vi "Aero_tunnel_monitor.vi"() -> ()   [LabVIEW 2013]
uses:
  Controls/Post_Process.ctl
  <vilib>/Platform/TimedLoop/XDataNode/timing_clust.ctl
  <vilib>/Platform/TimedLoop/XDataNode/nitl_modes.ctl
  <vilib>/Platform/TimedLoop/XDataNode/wakeup.ctl
  ADAM Client/Sub VIs/ADAM Controls/Update_scan_value.ctl
  Globals/Meas_global.vi
  <vilib>/Platform/TimedLoop/XDataNode/XDataNode.xnode
  <vilib>/Platform/TimedLoop/XDataNode/XDNodeRunTimeDep.lvlib
panel:
  in  "Display Graph?":bool
  in  "Menu Ring":u16(ring) items=["Lift", "Pitch", "Drag", "Side", "Yaw", "Roll"]
  in  "Samples":i32=1000
  out "Waveform Chart":dbl[](graph)
  in  "Output Roll":bool
  out "Roll":string="0.0 Nm"
  in  "Output Yaw":bool
  out "Yaw":string="0.0 Nm"
  in  "Output Pitch":bool
  out "Pitch":string="0.0 Nm"
  in  "Output SF":bool
  out "SF":string="0.0 N"
  in  "Output Drag":bool
  out "Drag":string="0.0 N"
  in  "Output Lift":bool
  out "Lift":string="0.0 N"
  in  "Balance Safety limits":T1(array[cluster])=[{"Max +ve Range"=80, "Max -ve Range"=80, "Axis"="Lift"}, {"Max +ve Range"=80, "Max -ve Range"=80, "Axis"="Pitch"}, {"Max +ve Range"=80, "Max -ve Range"=80, "Axis"="Drag"}, {"Max +ve Range"=80, "Max -ve Range"=80, "Axis"="Side-Force"}, {"Max +ve Range"=99, "Max -ve Range"=99, "Axis"="Yaw"}, {"Max +ve Range"=80, "Max -ve Range"=80, "Axis"="Roll"}] {"Max -ve Range" min=0 max=125; "Max +ve Range" min=0 max=125}
  out "Monitor Speed (Hz)":dbl
  out "Belt slip warning":bool
  out "Road Status":string="???"
  in  "GotoYaw":bool
  in  "NewYawPos":dbl
  out "YAW POSITION":dbl
  out "Required WindSpeedRatio":dbl
  out "ROAD SPEED m/s":dbl
  in  "BL Fan1":i32
  in  "BL Fan2":i32
  in  "Stop drive":bool
  in  "Start Drive":bool
  in  "Synch to Wind":bool
  out "Road Info":string="???"
  in  "stop":bool
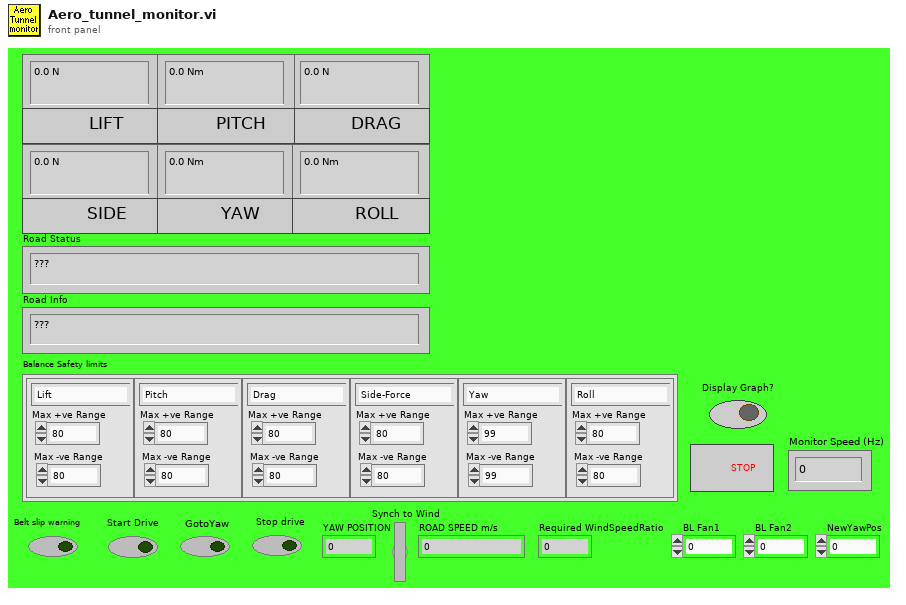
[diagram p1: front panel]
types:
  T1 = cluster{"Max +ve Range":i32, "Max -ve Range":i32, "Axis":string}[]
  T2 = typedef "Post_Process.ctl" = enum16{"Take New Data", "Post Process Raw Data File"}
  T3 = typedef "XDNodeRunTimeDep.lvlib/timing_clust.ctl" = cluster{"Expected End [f-1]":u64, "Actual End [f-1]":u64, "Finished Late? [f-1]":bool, "Expected End [i-1]":u64, "Actual End [i-1]":u64, "Finished Late? [i-1]":bool, "Expected Start [i]":u64, "Actual Start [i]":u64, "Expected Start [f]":u64, "Actual Start [f]":u64, "Source Name":string, "Structure Name":string, "Period":i64, "Deadline":i64, "Offset":i64, "Start":i64, "Priority":i32, "Timeout":i32, "Mode":T4, "Wakeup Reason":T5, "Error":errorcluster, "Source Type":string, "Secondary Source Type":string, "Global End Time":u64, "Global Start Time":u64, "Frame Duration":u64, "Iteration Duration":u64, "Assigned CPU":i32, "I/O Scan Engine Mode":u32}
  T4 = typedef "XDNodeRunTimeDep.lvlib/nitl_modes.ctl" = enum32{"No Change", "Process missed periods, maintain original phase", "Discard missed periods, maintain original phase", "Process missed periods, ignore original phase", "Discard missed periods, ignore original phase"}
  T5 = typedef "XDNodeRunTimeDep.lvlib/wakeup.ctl" = enum32{"Normal", "Aborted", "Asynchronous wakeup", "Timing source error", "Timed loop error", "Timeout"}
  T6 = typedef "Update_scan_value.ctl" = cluster{"Channel Name":string, "New Value":dbl}
  T7 = cluster{"Max +ve Range":i32, "Max -ve Range":i32, "Axis":string}
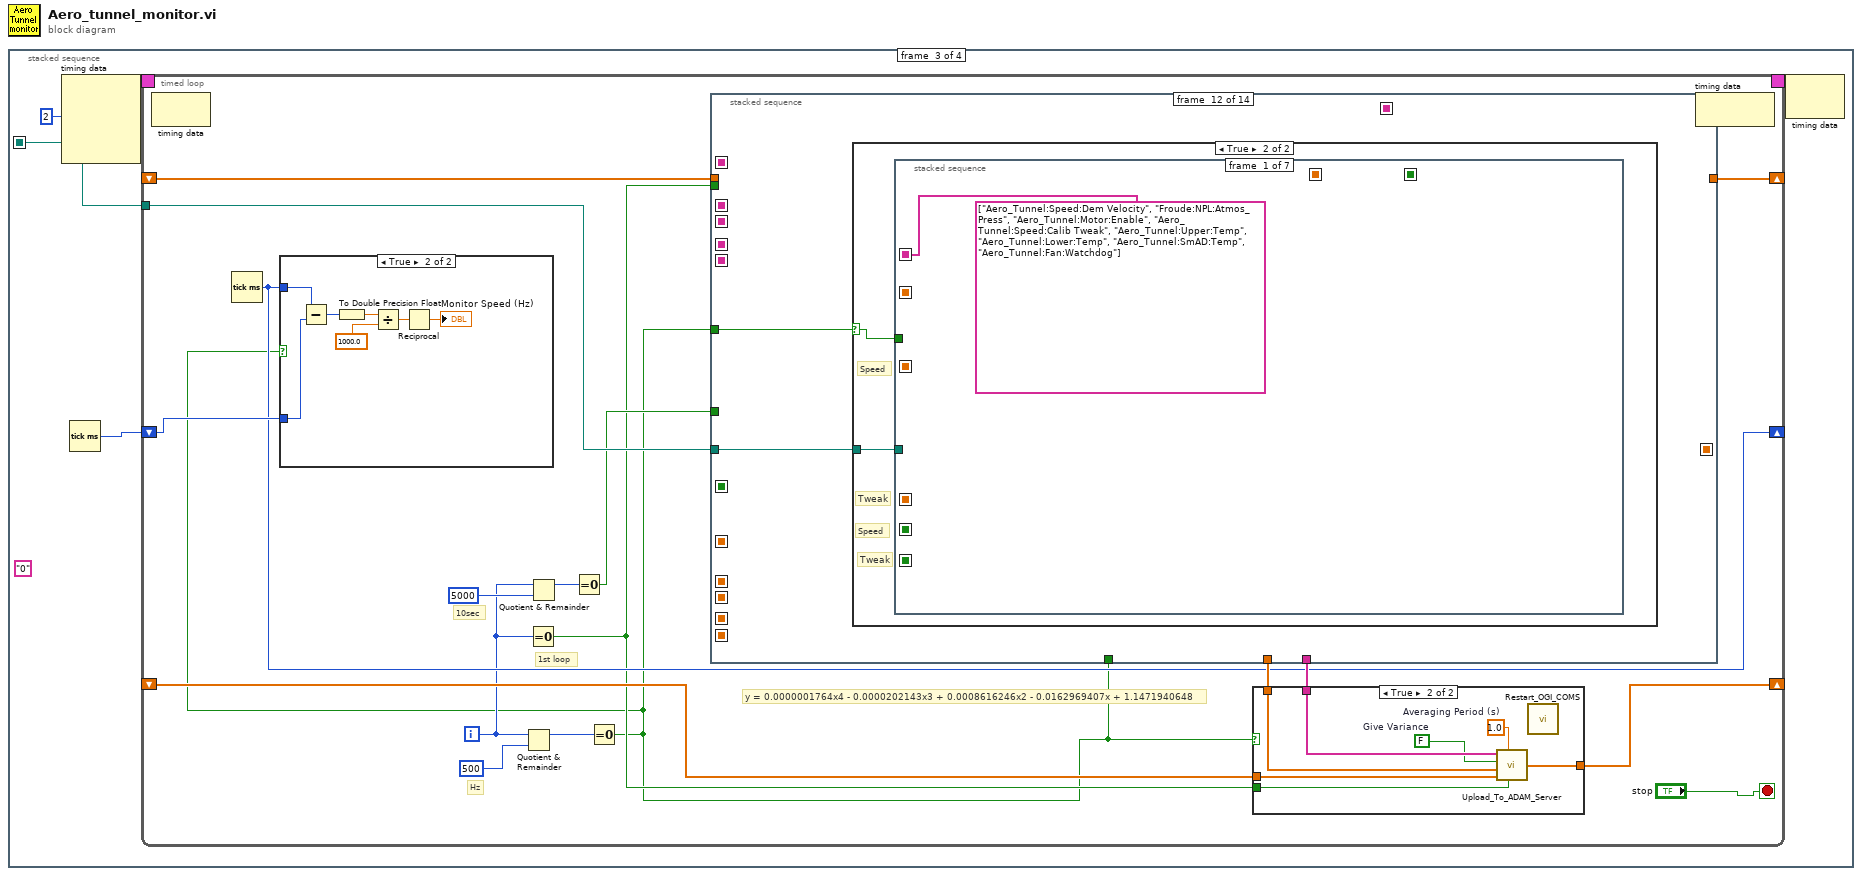
[diagram p0: block diagram]
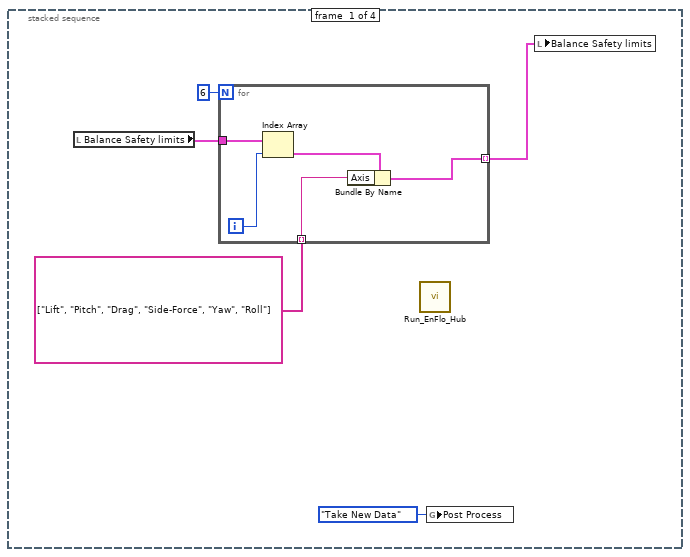
[diagram p2: hidden frame]
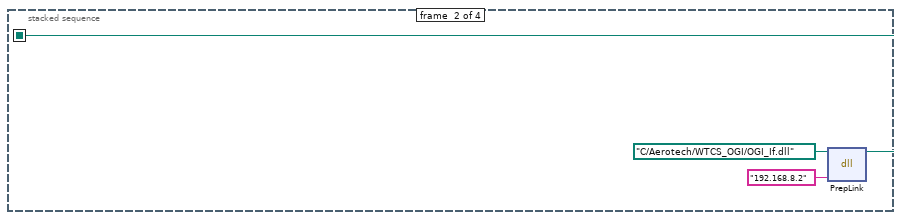
[diagram p3: hidden frame]
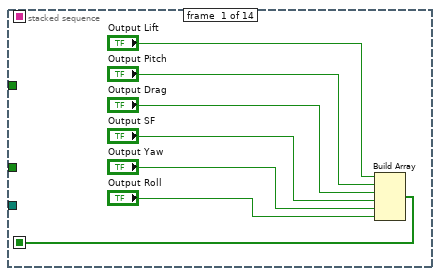
[diagram p6: hidden frame]
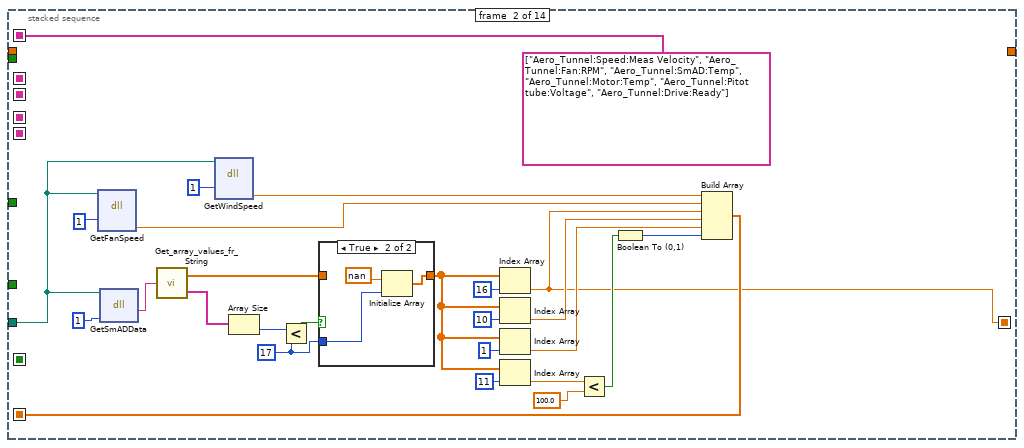
[diagram p7: hidden frame]
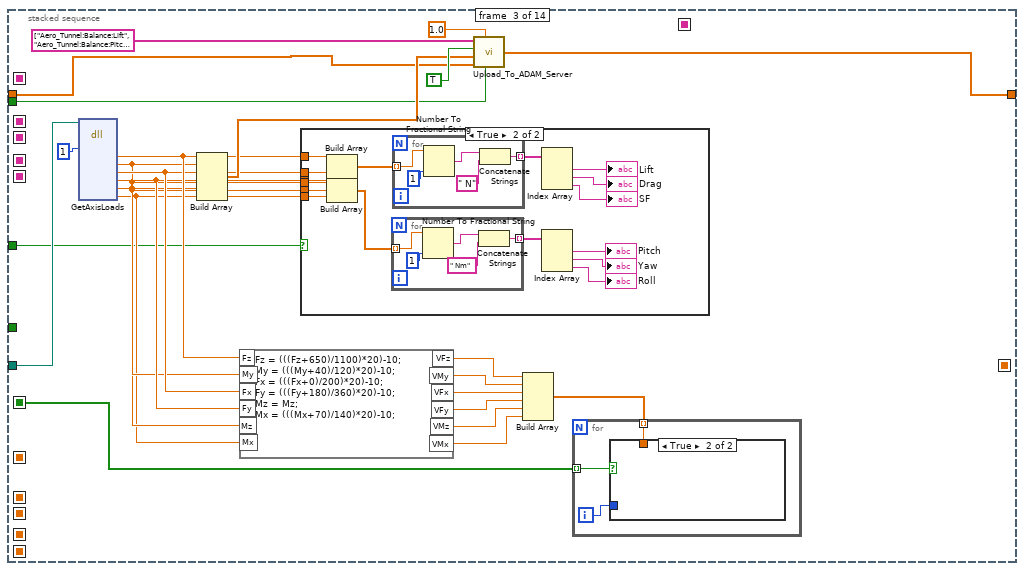
[diagram p9: hidden frame]
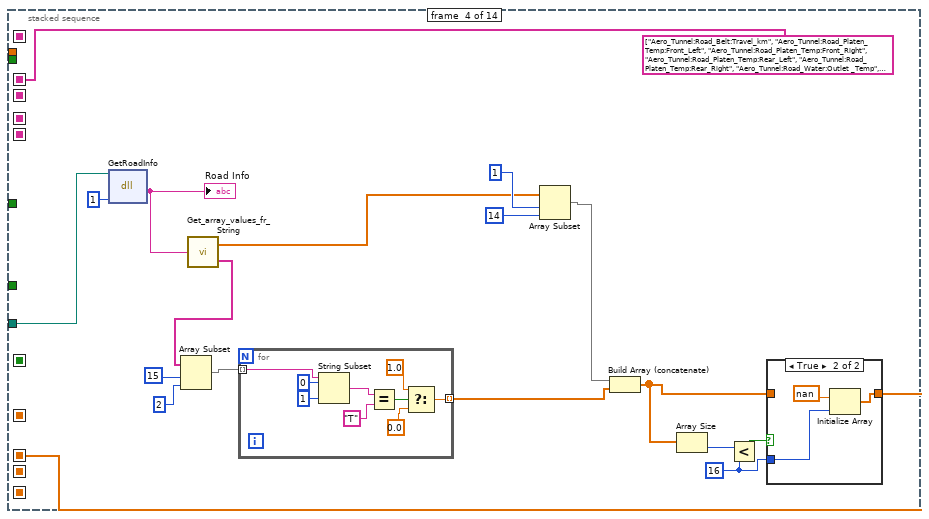
[diagram p12: hidden frame]
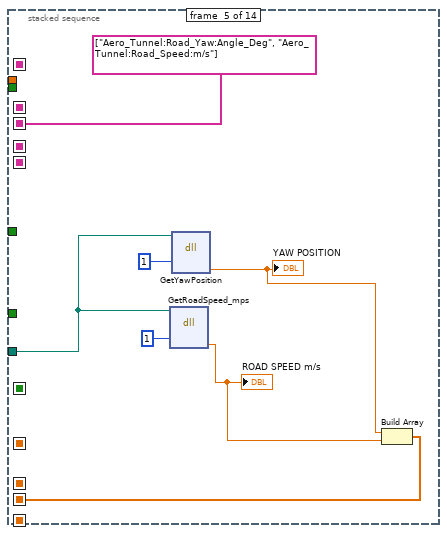
[diagram p14: hidden frame]
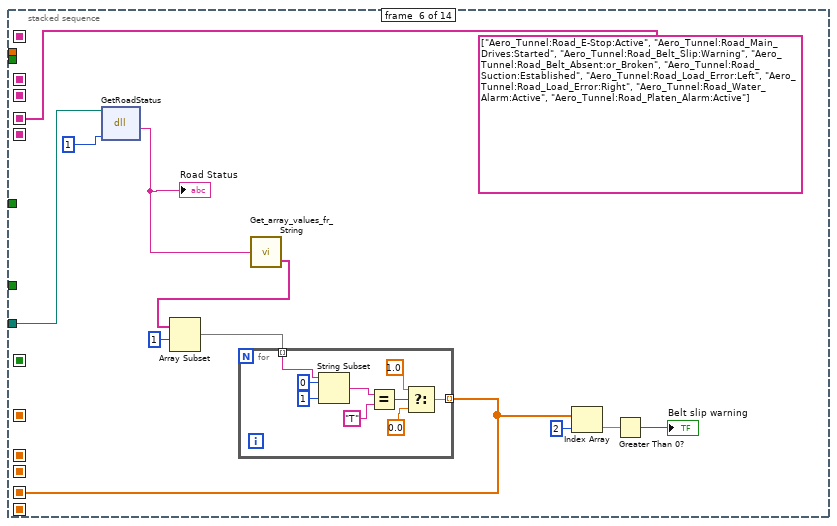
[diagram p15: hidden frame]
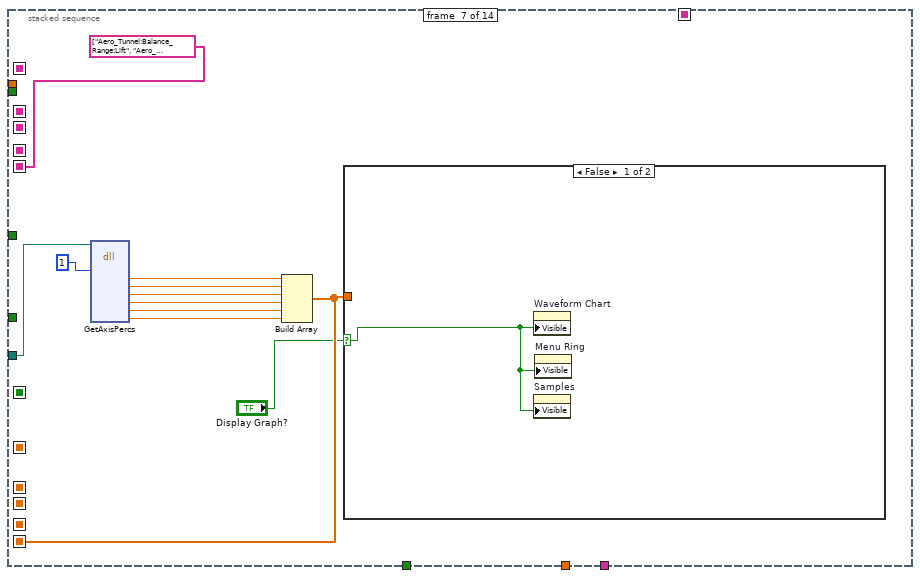
[diagram p16: hidden frame]
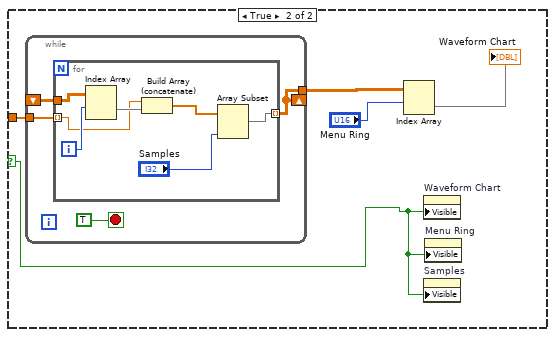
[diagram p17: hidden frame]
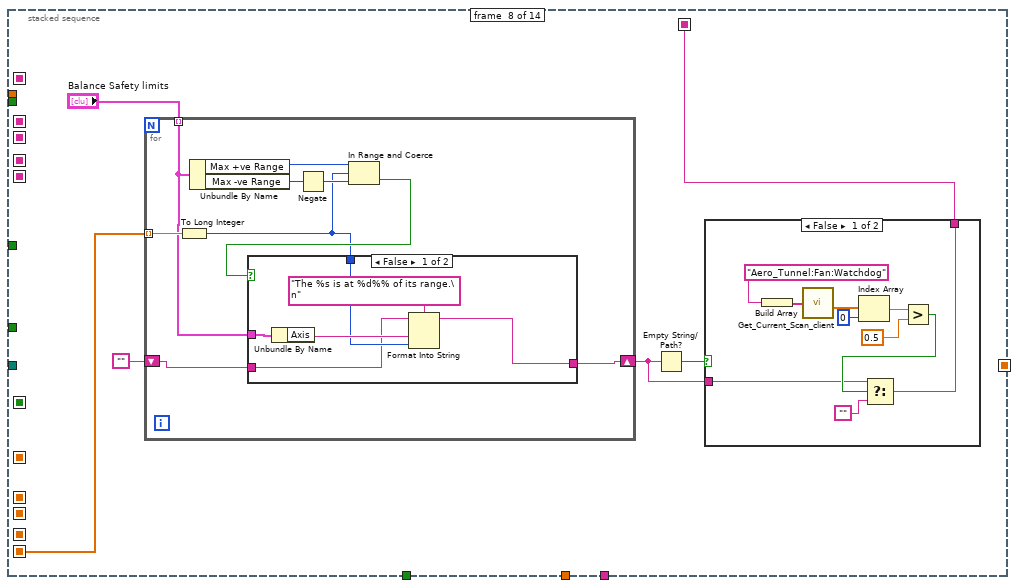
[diagram p18: hidden frame]
diagram:
  n1 = stacked-sequence {
    seq-local: [_ w11 _ _] -> [_ _ w18 w519]
    frame #0 {
      n2 = local read "Balance Safety limits"() -> (w4:T1)
      n3 = for {
        N: 6 -> [_]
        tunnel: w4 -> [w10]
        tunnel: [w7] -> w3 mode=indexing
        tunnel: string[] ["Lift", "Pitch", "Drag", "Side-Force", "Yaw", "Roll"] ("Channel Names") -> [w6] mode=indexing
        i -> [w9]
        n4 = Index Array(array=w10, index=w9) -> (element=w8:T7)
        n5 = Bundle By Name(cluster=w8, "Axis"=w6) -> (w7:T7)
      }
      n6 = call "Run_EnFlo_Hub.vi"() -> ()  [unwired: 8 in]
      n7 = global write "Meas_global.vi" "Post Process"(Post_Process."Take New Data" ("Post Process")) -> ()
      n8 = local write "Balance Safety limits"(w3) -> ()
    }
    frame #1 {
      n9 = dll-call lib="C:/Aerotech/Drivers/OGI_IF.dll" fn="PrepLink"(path in=path "C:/Aerotech/WTCS_OGI/OGI_If.dll", "IPAddress"="192.168.8.2") -> (path out=w11:path)  [unwired: 2 in, 3 out]
    }
    frame #2 {
      (unwired) "0" ("Channels")
      n10 = node-c288(i64 2 ("Period")) -> (w16:T3)  [unwired: 3 in]
      n11 = Tick Count (ms)() -> (millisecond timer value=w17:u32)
      n12 = timed-loop {
        shift-right: [w36] -> _
        shift-left: _ -> [w34]
        tunnel: w18 -> [w32]
        shift-right: [w30] -> _
        shift-left: _ -> [w31]
        timing: w16 -> [_]
        timing-out: [_] -> w15
        shift-right: [w28] -> _
        shift-left: w17 -> [w29]
        i -> [w22]
        stop <- "stop" stop-if-true
        # "1st loop"
        # "10sec"
        # "Hz"
        # "y = 0.0000001764x4 - 0.0000202143x3 + 0.0008616246x2 - 0.0162969407x + 1.1471940648"
        n13 = node-c288() -> ()  [unwired: 1 in, 1 out]
        n14 = Tick Count (ms)() -> (millisecond timer value=w28:u32)
        n15 = Quotient & Remainder(x=w22, y=500) -> (x-y*floor(x/y)=w25:i32)  [unwired: 1 out]
        n16 = Equal To 0?(x=w22) -> (x = 0?=w21:bool)
        n17 = Quotient & Remainder(x=w22, y=5000) -> (x-y*floor(x/y)=w24:i32)  [unwired: 1 out]
        n18 = Equal To 0?(x=w24) -> (x = 0?=w23:bool)
        n19 = Equal To 0?(x=w25) -> (x = 0?=w20:bool)
        n20 = case shown="True" w20 {
          tunnel: w29 -> [_ w43]
          tunnel: w28 -> [_ w42]
          frame False {
          }
          frame True {
            n21 = Subtract(x=w42, y=w43) -> (x-y=w41:u32)
            n22 = To Double Precision Float(number=w41) -> (double precision float=w37:dbl)
            n23 = Divide(x=w37, y=1000.0) -> (x/y=w39:dbl)
            n24 = Reciprocal(x=w39) -> (1/x=→"Monitor Speed (Hz)":dbl)
          }
        }
        n25 = stacked-sequence {
          seq-local: [_ string[] ["Aero_Tunnel:Speed:Meas Velocity", "Aero_Tunnel:Fan:RPM", "Aero_Tunnel:SmAD:Temp", "Aero_Tunnel:Motor:Temp", "Aero_Tunnel:Pitot tube:Voltage", "Aero_Tunnel:Drive:Ready"] ("Channel Names") _ _ _ _ _ _ _ _ _ _ _ _] -> [_ _ _ _ _ _ _ _ _ _ w319 _ _ _]
          seq-local: [_ w76 _ _ _ _ _ _ _ _ _ _ _ _] -> [_ _ _ _ _ _ _ _ _ _ w318 _ _ _]
          seq-local: [_ _ _ w144 _ _ _ _ _ _ _ _ _ _] -> [_ _ _ _ _ _ _ _ _ _ w315 _ _ _]
          seq-local: [_ _ _ string[] ["Aero_Tunnel:Road_Belt:Travel_km", "Aero_Tunnel:Road_Platen_Temp:Front_Left", "Aero_Tunnel:Road_Platen_Temp:Front_Right", "Aero_Tunnel:Road_Platen_Temp:Rear_Left", "Aero_Tunnel:Road_Platen_Temp:Rear_Right", "Aero_Tunnel:Road_Water:Outlet _Temp", "Aero_Tunnel:Road_Water:Inlet _Temp", "Aero_Tunnel:Road_Suction:Front", "Aero_Tunnel:Road_Suction:Middle", "Aero_Tunnel:Road_Suction:Rear", "Aero_Tunnel:Road_BL_Suction:Primary", "Aero_Tunnel:Road_BL_Suction:Secondary", "Aero_Tunnel:Road_LoadCell:Left", "Aero_Tunnel:Road_LoadCell:Right", "Aero_Tunnel:Road_Water_High:Temp_Alarm", "Aero_Tunnel:Road_Platen_High:Temp_Alarm"] ("Channel Names") _ _ _ _ _ _ _ _ _ _] -> [_ _ _ _ _ _ _ _ _ _ w304 _ _ _]
          seq-local: [_ _ _ _ string[] ["Aero_Tunnel:Road_Yaw:Angle_Deg", "Aero_Tunnel:Road_Speed:m/s"] ("Channel Names") _ _ _ _ _ _ _ _ _] -> [_ _ _ _ _ _ _ _ _ _ w314 _ _ _]
          seq-local: [_ _ _ _ w175 _ _ _ _ _ _ _ _ _] -> [_ _ _ _ _ _ _ _ _ _ w313 _ _ _]
          seq-local: [_ _ _ _ _ string[] ["Aero_Tunnel:Road_E-Stop:Active", "Aero_Tunnel:Road_Main_Drives:Started", "Aero_Tunnel:Road_Belt_Slip:Warning", "Aero_Tunnel:Road_Belt_Absent:or_Broken", "Aero_Tunnel:Road_Suction:Established", "Aero_Tunnel:Road_Load_Error:Left", "Aero_Tunnel:Road_Load_Error:Right", "Aero_Tunnel:Road_Water_Alarm:Active", "Aero_Tunnel:Road_Platen_Alarm:Active"] ("Channel Names") _ _ _ _ _ _ _ _] -> [_ _ _ _ _ _ _ _ _ _ w309 _ _ _]
          seq-local: [_ _ _ _ _ w188 _ _ _ _ _ _ _ _] -> [_ _ _ _ _ _ _ _ _ _ w308 _ _ _]
          seq-local: [w54 _ _ _ _ _ _ _ _ _ _ _ _ _] -> [_ _ w106 _ _ _ _ _ _ _ _ _ _ _]
          seq-local: [_ _ _ _ _ _ string[] ["Aero_Tunnel:Balance_Range:Lift", "Aero_Tunnel:Balance_Range:Pitch", "Aero_Tunnel:Balance_Range:Drag", "Aero_Tunnel:Balance_Range:Side-Force", "Aero_Tunnel:Balance_Range:Yaw", "Aero_Tunnel:Balance_Range:Roll"] ("Channel Names") _ _ _ _ _ _ _] -> [_ _ _ _ _ _ _ _ _ _ w305 _ _ _]
          seq-local: [_ _ _ _ _ _ w203 _ _ _ _ _ _ _] -> [_ _ _ _ _ _ _ w234 _ _ w306 _ _ _]
          seq-local: [_ _ _ _ _ _ _ w230 _ _ _ _ _ _] -> [_ _ _ _ _ _ _ _ w264 w283 _ _ _ _]
          seq-local: [_ w61 _ _ _ _ _ _ _ _ _ _ _ _] -> [_ _ _ _ _ _ _ _ _ w282 _ _ _ _]
          tunnel: [_ _ _ _ _ _ _ _ _ _ w317 _ _ _] -> w35
          tunnel: [_ _ _ _ _ _ _ _ _ _ w316 _ _ _] -> w33
          tunnel: w32 -> [_ w68 w113 w160 w178 w191 w212 _ _ _ w307 w321 w428 w455]
          tunnel: w20 -> [_ _ _ _ _ _ _ _ _ _ _ _ _ _]
          tunnel: w31 -> [_ _ w100 _ _ _ _ _ _ _ _ _ _ _]
          tunnel: [_ _ w99 _ _ _ _ _ _ _ _ _ _ _] -> w30
          tunnel: w20 -> [_ _ w92 _ _ _ _ _ _ _ _ w320 _ w454]
          tunnel: w23 -> [_ _ _ _ _ _ _ _ w263 _ _ _ w427 _]
          tunnel: w21 -> [_ _ w91 _ _ _ _ _ _ _ _ _ _ _]
          frame #0 {
            n26 = Build Array("Output Lift", "Output Pitch", "Output Drag", "Output SF", "Output Yaw", "Output Roll") -> (w54:bool[])
          }
          frame #1 {
            w62 = 17 ("y")
            n27 = dll-call lib="C:/Aerotech/Drivers/OGI_IF.dll" fn="GetFanSpeed"(path in=w68, "Enable"=1) -> ("FanSpeedinRPM"=w70:dbl)  [unwired: 3 in, 4 out]
            n28 = dll-call lib="C:/Aerotech/Drivers/OGI_IF.dll" fn="GetSmADData"(path in=w68, "Enable"=1) -> ("SmAD Data String"=w73:string)  [unwired: 2 in, 3 out]
            n29 = call "Get_array_values_fr_String.vi"("String Value"=w73) -> ("Numeric Array"=w63:dbl[], "String array"=w66:string[])
            n30 = dll-call lib="C:/Aerotech/Drivers/OGI_IF.dll" fn="GetWindSpeed"(path in=w68, "Enable"=1) -> ("Windspeed_M/s"=w69:dbl)  [unwired: 3 in, 4 out]
            n31 = Array Size(array=w66) -> (size(s)=w67:i32)
            n32 = Less?(x=w67, y=w62) -> (x < y?=w65:bool)
            n33 = case shown="True" w65 {
              tunnel: [w87 w90] -> w64
              tunnel: w63 -> [w87 _]
              tunnel: w62 -> [_ w88]
              frame False {
              }
              frame True {
                n34 = Initialize Array(nan, w88) -> (w90:dbl[])
              }
            }
            n35 = Index Array(array=w64, index=16) -> (element=w61:dbl)
            n36 = Index Array(array=w64, index=10) -> (element=w84:dbl)
            n37 = Index Array(array=w64, index=1) -> (element=w82:dbl)
            n38 = Index Array(array=w64, index=11) -> (element=w80:dbl)
            n39 = Less?(x=w80, y=100.0) -> (x < y?=w78:bool)
            n40 = Boolean To (0,1)(Boolean=w78) -> (0, 1=w77:i16)
            n41 = Build Array(w69, w70, w61, w84, w82, w77) -> (w76:dbl[])
          }
          frame #2 {
            n42 = dll-call lib="C:/Aerotech/Drivers/OGI_IF.dll" fn="GetAxisLoads"(path in=w113, "Enable"=1) -> ("Lift"=w98:dbl, "Pitch"=w95:dbl, "Drag"=w97:dbl, "side"=w96:dbl, "Yaw"=w94:dbl, "Roll"=w93:dbl)  [unwired: 3 in, 9 out]
            n43 = Build Array(w98, w95, w97, w96, w94, w93) -> (w101:dbl[])
            n44 = formula code="VFz = (((Fz+650)/1100)*20)-10;\nVMy = (((My+40)/120)*20)-10;\nVFx = (((Fx+0)/200)*20)-10;\nVFy = (((Fy+180)/360)*20)-10;\nVMz = Mz;\nVMx = (((Mx+70)/140)*20)-10;"("Fz"=w98, "My"=w95, "Fx"=w97, "Fy"=w96, "Mz"=w94, "Mx"=w93) -> ("VFz"=w112:dbl, "VMy"=w111:dbl, "VFx"=w110:dbl, "VFy"=w109:dbl, "VMz"=w108:dbl, "VMx"=w107:dbl)
            n45 = case shown="True" w92 {
              tunnel: w98 -> [_ w130]
              tunnel: w97 -> [_ w129]
              tunnel: w96 -> [_ w128]
              tunnel: w95 -> [_ w122]
              tunnel: w94 -> [_ w121]
              tunnel: w93 -> [_ w120]
              frame False {
              }
              frame True {
                n46 = Build Array(w130, w129, w128) -> (w127:dbl[])
                n47 = Build Array(w122, w121, w120) -> (w119:dbl[])
                n48 = for {
                  tunnel: w119 -> [w131] mode=indexing
                  tunnel: [w135] -> w118 mode=indexing
                  n49 = Number To Fractional String(number=w131, precision (6)=i16 1) -> (F-format string=w132:string)  [unwired: 2 in]
                  n50 = Concatenate Strings(w132, " Nm" ("string")) -> (w135:string)
                }
                n51 = for {
                  tunnel: w127 -> [w136] mode=indexing
                  tunnel: [w140] -> w126 mode=indexing
                  n52 = Number To Fractional String(number=w136, precision (6)=i16 1) -> (F-format string=w137:string)  [unwired: 2 in]
                  n53 = Concatenate Strings(w137, " N" ("string")) -> (w140:string)
                }
                n54 = Index Array(array=w126) -> (element #1=→"Lift":string, element #2=→"Drag":string, element #3=→"SF":string)  [unwired: 3 in]
                n55 = Index Array(array=w118) -> (element #1=→"Pitch":string, element #2=→"Yaw":string, element #3=→"Roll":string)  [unwired: 3 in]
              }
            }
            n56 = call "Upload_To_ADAM_Server.vi"("First Loop"=w91, "Averaging Period (s)"=1.0, "Shift In"=w100, "Channel Values"=w101, "Give Variance"=TRUE, "Channel Names"=string[] ["Aero_Tunnel:Balance:Lift", "Aero_Tunnel:Balance:Pitch", "Aero_Tunnel:Balance:Drag", "Aero_Tunnel:Balance:Side-Force", "Aero_Tunnel:Balance:Yaw", "Aero_Tunnel:Balance:Roll"]) -> ("Shift Out"=w99:dbl[])
            n57 = Build Array(w112, w111, w110, w109, w108, w107) -> (w105:dbl[])
            n58 = for {
              tunnel: w106 -> [w143] mode=indexing
              tunnel: w105 -> [w142] mode=indexing
              i -> [w141]
              n59 = case shown="True" w143 {
                tunnel: w142 -> [_ _]
                tunnel: w141 -> [_ _]
                frame False {
                }
                frame True {
                }
              }
            }
          }
          frame #3 {
            w147 = 16 ("y")
            n60 = dll-call lib="C:/Aerotech/Drivers/OGI_IF.dll" fn="GetRoadInfo"(path in=w160, "Enable"=1) -> ("Road Info"=w159:string)  [unwired: 3 in, 2 out]
            "Road Info" <- w159
            n61 = call "Get_array_values_fr_String.vi"("String Value"=w159) -> ("Numeric Array"=w146:dbl[], "String array"=w150:string[])
            n62 = Array Subset(array=w150, index=15, length=2) -> (w154:string[])
            n63 = for {
              tunnel: w154 -> [w172] mode=indexing
              tunnel: [w166] -> w153 mode=indexing
              n64 = String Subset(string=w172, offset (0)=0, length (rest)=1 ("length (rest)")) -> (substring=w171:string)
              n65 = Equal?(x=w171, y="T") -> (x = y?=w169:bool)
              n66 = Select(t=1.0, s=w169, f=0.0) -> (s? t:f=w166:dbl)
            }
            n67 = Array Subset(array=w146, index=1, length=14) -> (w152:dbl[])
            n68 = Build Array (concatenate)(w152, w153) -> (w145:dbl[])
            n69 = Array Size(array=w145) -> (size(s)=w149:i32)
            n70 = Less?(x=w149, y=w147) -> (x < y?=w148:bool)
            n71 = case shown="True" w148 {
              tunnel: [w162 w165] -> w144
              tunnel: w145 -> [w162 _]
              tunnel: w147 -> [_ w163]
              frame False {
              }
              frame True {
                n72 = Initialize Array(nan, w163) -> (w165:dbl[])
              }
            }
          }
          frame #4 {
            n73 = dll-call lib="C:/Aerotech/Drivers/OGI_IF.dll" fn="GetRoadSpeed_mps"(path in=w178, "Enable"=1) -> ("RoadSpeed_mps"=w176:dbl)  [unwired: 3 in, 4 out]
            "ROAD SPEED m/s" <- w176
            n74 = dll-call lib="C:/Aerotech/Drivers/OGI_IF.dll" fn="GetYawPosition"(path in=w178, "Enable"=1) -> ("Yaw Position"=w177:dbl)  [unwired: 3 in, 4 out]
            "YAW POSITION" <- w177
            n75 = Build Array(w177, w176) -> (w175:dbl[])
          }
          frame #5 {
            n76 = dll-call lib="C:/Aerotech/Drivers/OGI_IF.dll" fn="GetRoadStatus"(path in=w191, "Enable"=1) -> ("Road Status"=w190:string)  [unwired: 3 in, 2 out]
            "Road Status" <- w190
            n77 = call "Get_array_values_fr_String.vi"("String Value"=w190) -> ("String array"=w184:string[])  [unwired: 1 out]
            n78 = Array Subset(array=w184, index=1) -> (w182:string[])  [unwired: 1 in]
            n79 = for {
              tunnel: [w194] -> w188 mode=indexing
              tunnel: w182 -> [w193] mode=indexing
              n80 = String Subset(string=w193, offset (0)=0, length (rest)=1 ("length (rest)")) -> (substring=w199:string)
              n81 = Equal?(x=w199, y="T") -> (x = y?=w197:bool)
              n82 = Select(t=1.0, s=w197, f=0.0) -> (s? t:f=w194:dbl)
            }
            n83 = Index Array(array=w188, index=2) -> (element=w186:dbl)
            n84 = Greater Than 0?(x=w186) -> (x > 0?=→"Belt slip warning":bool)
          }
          frame #6 {
            n85 = dll-call lib="C:/Aerotech/Drivers/OGI_IF.dll" fn="GetAxisPercs"(path in=w212, "Enable"=1) -> ("Lift"=w210:dbl, "Pitch"=w209:dbl, "Drag"=w208:dbl, "side"=w207:dbl, "Yaw"=w206:dbl, "Roll"=w205:dbl)  [unwired: 3 in, 9 out]
            n86 = Build Array(w210, w209, w208, w207, w206, w205) -> (w203:dbl[])
            n87 = case shown="False" "Display Graph?" {
              selector: "Display Graph?" -> [w213 w214]
              tunnel: w203 -> [_ w218]
              frame False {
                n88 = property on="Waveform Chart" class="WFChart (strict)"("Visible"=w213) -> ()  [unwired: 2 in, 2 out]
                n89 = property on="Samples" class="DigNum (strict)"("Visible"=w213) -> ()  [unwired: 2 in, 2 out]
                n90 = property on="Menu Ring" class="Ring (strict)"("Visible"=w213) -> ()  [unwired: 2 in, 2 out]
              }
              frame True {
                n91 = while {
                  shift-right: [w220] -> _
                  shift-left: _ -> [w222]
                  tunnel: w218 -> [w221]
                  tunnel: [w220] -> w217
                  stop <- TRUE stop-if-true
                  n92 = for {
                    tunnel: w222 -> [w225]
                    tunnel: w221 -> [w223] mode=indexing
                    tunnel: [w228] -> w220 mode=indexing
                    i -> [w226]
                    n93 = Index Array(array=w225, index (row)=w226) -> (element=w224:dbl[])  [unwired: 1 in]
                    n94 = Build Array (concatenate)(w223, w224) -> (w229:dbl[])
                    n95 = Array Subset(array=w229, length="Samples") -> (w228:dbl[])  [unwired: 1 in]
                  }
                }
                n96 = Index Array(array=w217, index (row)="Menu Ring") -> (element=→"Waveform Chart":dbl[])  [unwired: 1 in]
                n97 = property on="Waveform Chart" class="WFChart (strict)"("Visible"=w214) -> ()  [unwired: 2 in, 2 out]
                n98 = property on="Samples" class="DigNum (strict)"("Visible"=w214) -> ()  [unwired: 2 in, 2 out]
                n99 = property on="Menu Ring" class="Ring (strict)"("Visible"=w214) -> ()  [unwired: 2 in, 2 out]
              }
            }
          }
          frame #7 {
            n100 = for {
              tunnel: "Balance Safety limits" -> [w250] mode=indexing
              tunnel: w234 -> [w253] mode=indexing
              shift-right: [w247] -> w231
              shift-left: "" -> [w248]
              n101 = To Long Integer(number=w253) -> (32bit integer=w249:i32)
              n102 = Unbundle By Name(w250) -> ("Max +ve Range"=w255:i32, "Max -ve Range"=w254:i32)
              n103 = Negate(x=w254) -> (-x=w252:i32)
              n104 = In Range and Coerce(upper limit=w255, x=w249, lower limit=w252) -> (In Range?=w251:bool)  [unwired: 1 out]
              n105 = case shown="False" w251 {
                tunnel: w250 -> [w261 _]
                tunnel: w249 -> [w259 _]
                tunnel: w248 -> [w257 w262]
                tunnel: [w256 w262] -> w247
                frame False {
                  n106 = Unbundle By Name(w261) -> ("Axis"=w260:string)
                  n107 = Format Into String(format string="The %s is at %d%% of its range.\n", initial string=w257, w260, w259) -> (resulting string=w256:string)  [unwired: 1 in, 1 out]
                }
                frame True {
                }
              }
            }
            n108 = Empty String/Path?(string/path=w231) -> (empty?=w232:bool)
            n109 = case shown="False" w232 {
              tunnel: w231 -> [w238 w246]
              tunnel: [w236 w246] -> w230
              frame False {
                n110 = Build Array("Aero_Tunnel:Fan:Watchdog") -> (w245:string[])
                n111 = call "Get_Current_Scan_client.vi"("ADAM Ch Names"=w245) -> ("Numerical Values"=w243:dbl[])  [unwired: 1 in, 2 out]
                n112 = Index Array(array=w243, index=0) -> (element=w241:dbl)
                n113 = Greater?(x=w241, y=0.5) -> (0:w239:bool)
                n114 = Select(t=w238, s=w239, f="") -> (s? t:f=w236:string)
              }
              frame True {
              }
            }
          }
          frame #8 {
            n115 = while {
              tunnel: w264 -> [w268]
              tunnel: w263 -> [w265]
              stop <- TRUE stop-if-true
              n116 = Empty String/Path?(string/path=w268) -> (empty?=w270:bool)
              n117 = Not(x=w270) -> (.not. x?=w266:bool)
              n118 = Compound Arithmetic op=AND(w266, w265) -> (w269:bool)
              n119 = case shown="True" w269 {
                tunnel: w268 -> [_ w275]
                frame False {
                }
                frame True {
                  w274 = string[] ["Aero_Tunnel:Fan:Watchdog", "Aero_Tunnel:Road:Watchdog", "Aero_Tunnel:Speed:Dem Velocity", "Aero_Tunnel:OGI Dem:Speed"] ("Channel Names")
                  n120 = Format Into String(format string="The Aero Tunnel balance has gone outside of its limits.\n%s\nThe Aero_Tunnel:Fan:Watchdog has therefore been disabled. ", w275) -> (resulting string=w276:string)  [unwired: 2 in, 1 out]
                  n121 = Bundle By Name(cluster=errorcluster {"status"=TRUE, "code"=0, "source"=""} ("error in (no error)"), "source"=w276) -> (w278:errorcluster)
                  n122 = Array Size(array=w274) -> (size(s)=w273:i32)
                  n123 = call "EnFlo_Error_Handler.vi"("error in (no error)"=w278, "Error Type"="Aero Tunnel Balance Range Trip", "Dialog Box (T)"=FALSE) -> ()  [unwired: 3 out]
                  n124 = Initialize Array(0.0, w273) -> (w271:dbl[])
                  n125 = call "ASYNC_Adam_client.vi"("Values"=w271, "Channel Names"=w274) -> ()  [unwired: 2 out]
                }
              }
            }
          }
          frame #9 {
            n126 = while {
              tunnel: w283 -> [_]
              shift-right: [w288] -> _
              shift-left: _ -> [w287]
              tunnel: w282 -> [w285]
              stop <- TRUE stop-if-true
              n127 = Greater?(x=w285, y=35.0) -> (0:w288:bool)
              n128 = Number To Fractional String(number=w285, precision (6)=i16 2) -> (F-format string=w284:string)  [unwired: 2 in]
              n129 = Compound Arithmetic op=AND(invert w287, w288) -> (w291:bool)
              n130 = case shown="True" w291 {
                tunnel: w284 -> [_ w296]
                frame False {
                }
                frame True {
                  w295 = string[] ["Aero_Tunnel:Fan:Watchdog", "Aero_Tunnel:Road:Watchdog", "Aero_Tunnel:Speed:Dem Velocity", "Aero_Tunnel:OGI Dem:Speed"] ("Channel Names")
                  n131 = Format Into String(format string="The Aero Tunnel temperature has gone above it's limits and is:\n%s\nThe Aero_Tunnel:Fan:Watchdog has therefore been disabled. ", w296) -> (resulting string=w297:string)  [unwired: 2 in, 1 out]
                  n132 = Bundle By Name(cluster=errorcluster {"status"=TRUE, "code"=0, "source"=""} ("error in (no error)"), "source"=w297) -> (w299:errorcluster)
                  n133 = Array Size(array=w295) -> (size(s)=w294:i32)
                  n134 = call "EnFlo_Error_Handler.vi"("error in (no error)"=w299, "Error Type"="Aero Tunnel Temperature Trip", "Dialog Box (T)"=FALSE) -> ()  [unwired: 3 out]
                  n135 = Initialize Array(0.0, w294) -> (w292:dbl[])
                  n136 = call "ASYNC_Adam_client.vi"("Values"=w292, "Channel Names"=w295) -> ()  [unwired: 2 out]
                }
              }
            }
          }
          frame #10 {
            n137 = Build Array (concatenate)(w318, w315, w313, w308, w306) -> (w317:dbl[])
            n138 = Boolean To (0,1)(Boolean="GotoYaw") -> (0, 1=w312:i16)
            n139 = Build Array (concatenate)(w319, w304, w314, w309, w305) -> (w316:string[])
            n140 = To Long Integer(number=w312) -> (32bit integer=w303:i32)
            n141 = dll-call lib="C:/Aerotech/Drivers/OGI_IF.dll" fn="GotoYawPosition"(path in=w307, "Enable"=w303, "NewYawPos"="NewYawPos") -> ()  [unwired: 3 in, 4 out]
          }
          frame #11 {
            n142 = case shown="True" w320 {
              selector: w320 -> [_ w322]
              tunnel: w321 -> [_ w323]
              frame False {
              }
              frame True {
                # "Tweak"
                # "Speed"
                # "Tweak"
                # "Speed"
                n143 = stacked-sequence {
                  seq-local: [_ w337 _ _ _ _ _] -> [_ _ _ w377 w391 _ w414]
                  seq-local: [_ w328 _ _ _ _ _] -> [_ _ _ w376 w388 _ _]
                  seq-local: [_ w335 _ _ _ _ _] -> [_ _ _ _ _ w403 _]
                  seq-local: [_ w331 _ _ _ _ _] -> [_ _ _ _ _ _ w416]
                  seq-local: [_ w329 _ _ _ _ _] -> [_ _ _ _ w389 _ _]
                  seq-local: [_ w327 _ _ _ _ _] -> [_ _ _ _ w387 _ _]
                  seq-local: [string[] ["Aero_Tunnel:Speed:Dem Velocity", "Froude:NPL:Atmos_Press", "Aero_Tunnel:Motor:Enable", "Aero_Tunnel:Speed:Calib Tweak", "Aero_Tunnel:Upper:Temp", "Aero_Tunnel:Lower:Temp", "Aero_Tunnel:SmAD:Temp", "Aero_Tunnel:Fan:Watchdog"] ("appended array") _ _ _ _ _ _] -> [_ w326 _ _ _ _ _]
                  seq-local: [_ w325 _ _ _ _ _] -> [_ _ w361 _ _ _ _]
                  tunnel: w323 -> [_ w339 _ w375 w390 w402 w417]
                  tunnel: w322 -> [_ _ _ _ _ _ w412]
                  frame #0 {
                  }
                  frame #1 {
                    n144 = call "Get_Current_Scan_client.vi"("ADAM Ch Names"=w326) -> ("Numerical Values"=w325:dbl[])  [unwired: 1 in, 2 out]
                    n145 = Index Array(array=w325, index=0) -> (element=w337:dbl)
                    n146 = Index Array(array=w325, index=3) -> (element=w329:dbl)
                    n147 = Index Array(array=w325, index=1) -> (element=w335:dbl)
                    n148 = while {
                      tunnel: w339 -> [w347]
                      tunnel: w337 -> [w346]
                      shift-right: [w346] -> _
                      shift-left: _ -> [w345]
                      shift-right: [w342] -> _
                      shift-left: _ -> [w343]
                      tunnel: w329 -> [w342]
                      tunnel: [w341] -> w328
                      tunnel: [w340] -> w327
                      stop <- TRUE stop-if-true
                      n149 = Not Equal?(x=w346, y=w345) -> (x != y?=w341:bool)
                      n150 = Not Equal?(x=w342, y=w343) -> (x != y?=w340:bool)
                      n151 = case shown="True" w341 {
                        tunnel: w347 -> [_ w348]
                        tunnel: w346 -> [_ w349]
                        frame False {
                        }
                        frame True {
                          n152 = Greater?(x=w349, y=0.2) -> (0:w350:bool)
                          n153 = Boolean To (0,1)(Boolean=w350) -> (0, 1=w353:i16)
                          n154 = dll-call lib="C:/Aerotech/Drivers/OGI_IF.dll" fn="SetFanSystemState"(path in=w348, "Enable"=1, "Fan ONOFF"=w353) -> ()  [unwired: 3 in, 4 out]
                        }
                      }
                    }
                    n155 = Index Array(array=w325, index=2) -> (element=w333:dbl)
                    n156 = Greater?(x=w333, y=0.5) -> (0:w331:bool)
                  }
                  frame #2 {
                    # "allowed temp."
                    n157 = Index Array(array=w361, index=7) -> (element=w359:dbl)
                    n158 = Array Subset(array=w361, index=4, length=3) -> (w363:dbl[])
                    n159 = Array Max & Min(array=w363) -> (max value=w354:dbl)  [unwired: 3 out]
                    n160 = Greater?(x=w359, y=0.5) -> (0:w356:bool)
                    n161 = Greater?(x=w354, y=35.0) -> (0:w357:bool)
                    n162 = And(x=w357, y=w356) -> (x .and. y?=w355:bool)
                    n163 = case shown="True" w355 {
                      tunnel: w354 -> [_ w368]
                      frame False {
                      }
                      frame True {
                        n164 = Format Into String(format string="Aero Tunnel temp is %.1f. The Aero_Tunnel:Fan:Watchdog has therefore been disabled. ", w368) -> (resulting string=w366:string)  [unwired: 2 in, 1 out]
                        n165 = Bundle By Name(cluster=errorcluster {"status"=TRUE, "code"=0, "source"=""} ("error in (no error)"), "source"=w366) -> (w369:errorcluster)
                        n166 = call "EnFlo_Error_Handler.vi"("error in (no error)"=w369, "Error Type"="Aero Tunnel over temp", "Dialog Box (T)"=FALSE) -> ()  [unwired: 3 out]
                        n167 = call "ASYNC_Adam_client.vi"("Values"=dbl[] [0.0, 0.0], "Channel Names"=string[] ["Aero_Tunnel:Fan:Watchdog", "Aero_Tunnel:Road:Watchdog"]) -> ()  [unwired: 2 out]
                      }
                    }
                  }
                  frame #3 {
                    n168 = case shown="True" w376 {
                      tunnel: w377 -> [_ w384]
                      tunnel: w375 -> [_ w385]
                      frame False {
                      }
                      frame True {
                        n169 = call "Polynomial_convert.vi"("Calib constants"=dbl[] [1.1471940648, -0.0162969407, 0.0008616246, -2.02143e-05, 1.764e-07], "Voltage"=w384) -> ("Eng Values"=w381:dbl)  [unwired: 4 in]
                        n170 = In Range and Coerce(upper limit=1.12, x=w381, lower limit=0.88) -> (coerced(x)=w378:dbl)  [unwired: 1 out]
                        "Required WindSpeedRatio" <- w378
                        n171 = dll-call lib="C:/Aerotech/Drivers/OGI_IF.dll" fn="SetWindSpeedRatio"(path in=w385, "Enable"=1 ("t"), "Required WindSpeedRatio"=w378) -> ()  [unwired: 4 in, 3 out]
                      }
                    }
                  }
                  frame #4 {
                    n172 = Or(x=w388, y=w387) -> (x .or. y?=w386:bool)
                    n173 = case shown="True" w386 {
                      tunnel: w391 -> [_ w396]
                      tunnel: w390 -> [_ w394]
                      tunnel: w389 -> [_ w397]
                      frame False {
                      }
                      frame True {
                        n174 = Divide(x=w397, y=100.0) -> (x/y=w399:dbl)
                        n175 = Increment(x=w399) -> (x+1=w400:dbl)
                        n176 = Multiply(x=w400, y=w396) -> (x*y=w395:dbl)
                        n177 = call "Polynomial_convert.vi"("Calib constants"=dbl[] [36.127, 22.861], "Voltage"=w395) -> ("Eng Values"=w393:dbl)  [unwired: 4 in]
                        n178 = dll-call lib="C:/Aerotech/Drivers/ATE_Surrey_WTCS.dll" fn="SetFanspeed"(path in=w394, "Enable"=1 ("t"), "NewFanSpeed"=w393) -> ()  [unwired: 3 in, 4 out]
                      }
                    }
                  }
                  frame #5 {
                    n179 = while {
                      shift-right: [w405] -> _
                      shift-left: _ -> [w408]
                      tunnel: w403 -> [w405]
                      tunnel: w402 -> [w406]
                      stop <- TRUE stop-if-true
                      n180 = Equal?(x=w405, y=w408) -> (x = y?=w407:bool)
                      n181 = case shown="True" w407 {
                        tunnel: w406 -> [_ w411]
                        tunnel: w405 -> [_ w409]
                        frame False {
                        }
                        frame True {
                          n182 = dll-call lib="C:/Aerotech/Drivers/OGI_IF.dll" fn="SetNewbaroPr_mB"(path in=w411, "Enable"=1, "NewPressure"=w409) -> ()  [unwired: 3 in, 4 out]
                        }
                      }
                    }
                  }
                  frame #6 {
                    n183 = Greater?(x=w414, y=0.1) -> (0:w413:bool)
                    n184 = while {
                      shift-right: [w422] -> _
                      shift-left: _ -> [w421]
                      tunnel: w416 -> [w422]
                      tunnel: w417 -> [w424]
                      tunnel: w413 -> [w420]
                      tunnel: w412 -> [w418]
                      stop <- TRUE stop-if-true
                      n185 = Compound Arithmetic op=AND(w422, invert w421, w420, w418) -> (w419:bool)
                      n186 = case shown="True" w419 {
                        tunnel: w424 -> [_ w426]
                        frame False {
                        }
                        frame True {
                          n187 = dll-call lib="C:/Aerotech/Drivers/OGI_IF.dll" fn="SetPitotZero"(path in=w426, "Enable"=1) -> ()  [unwired: 2 in, 4 out]
                        }
                      }
                    }
                  }
                }
              }
            }
          }
          frame #12 {
            n188 = while {
              tunnel: w428 -> [w435]
              shift-right: [w433] -> _
              shift-left: _ -> [w432]
              tunnel: w427 -> [w431]
              shift-right: [w429] -> _
              shift-left: _ -> [w430]
              stop <- TRUE stop-if-true
              # "Do every 10 seconds"
              n189 = case shown="True" w431 {
                tunnel: w435 -> [_ _]
                tunnel: [w437 w451] -> w433
                tunnel: w432 -> [w437 w450]
                tunnel: w430 -> [w436 w442]
                tunnel: [w436 w440] -> w429
                frame False {
                  (unwired) FALSE
                }
                frame True {
                  # "Do every 10 minutes"
                  # "flip flop every 10 cycles"
                  n190 = Increment(x=w442) -> (x+1=w439:i32)
                  n191 = Greater?(x=w439, y=60) -> (0:w438:bool)
                  n192 = case shown="True" w438 {
                    tunnel: [w452 0] -> w440
                    tunnel: w439 -> [w452 _]
                    frame False {
                    }
                    frame True {
                    }
                  }
                  n193 = Select(t=1.0, s=w450, f=0.0) -> (s? t:f=w444:dbl)
                  n194 = Bundle By Name(cluster=T6 {"Channel Name"="Aero_Tunnel:Server:Pulse", "New Value"=0.0} ("Update Scan Value Cluster"), "New Value"=w444) -> (w446:T6)
                  n195 = Not(x=w450) -> (.not. x?=w451:bool)
                  n196 = Build Array(w446) -> (w445:T6[])
                  n197 = call "Update_Current_Value_client.vi"("Don't Bother with check?"=TRUE, "Update array in"=w445) -> ()
                }
              }
            }
          }
          frame #13 {
            n198 = while {
              shift-right: [w466] -> _
              shift-left: _ -> [w468]
              tunnel: w454 -> [w467]
              tunnel: w455 -> [w464]
              shift-right: [w462] -> _
              shift-left: _ -> [w463]
              shift-right: [w460] -> _
              shift-left: _ -> [w461]
              shift-right: [w457] -> _
              shift-left: _ -> [w459]
              shift-right: [w456] -> _
              shift-left: _ -> [w458]
              stop <- TRUE stop-if-true
              n199 = stacked-sequence {
                tunnel: w468 -> [w474 _ _ _]
                tunnel: w467 -> [w472 w484 w494 w506]
                tunnel: ["Synch to Wind" _ _ _] -> w466
                tunnel: w464 -> [w469 w482 w492 w508]
                tunnel: w463 -> [_ w481 _ _]
                tunnel: [_ "Start Drive" _ _] -> w462
                tunnel: w461 -> [_ _ w491 _]
                tunnel: [_ _ "Stop drive" _] -> w460
                tunnel: w459 -> [_ _ _ w505]
                tunnel: w458 -> [_ _ _ w502]
                tunnel: [_ _ _ "BL Fan1"] -> w457
                tunnel: [_ _ _ "BL Fan2"] -> w456
                frame #0 {
                  n200 = Not Equal?(x="Synch to Wind", y=w474) -> (x != y?=w473:bool)
                  n201 = Or(x=w473, y=w472) -> (x .or. y?=w470:bool)
                  n202 = case shown="True" w470 {
                    tunnel: "Synch to Wind" -> [_ w477]
                    tunnel: w469 -> [_ w476]
                    frame False {
                    }
                    frame True {
                      n203 = Boolean To (0,1)(Boolean=w477) -> (0, 1=w478:i16)
                      n204 = To Long Integer(number=w478) -> (32bit integer=w475:i32)
                      n205 = dll-call lib="C:/Aerotech/Drivers/OGI_IF.dll" fn="RoadSyncToWind"(path in=w476, "Enable"=1, "SynchState"=w475) -> ()  [unwired: 3 in, 4 out]
                    }
                  }
                }
                frame #1 {
                  n206 = Not Equal?(x="Start Drive", y=w481) -> (x != y?=w485:bool)
                  n207 = Or(x=w485, y=w484) -> (x .or. y?=w483:bool)
                  n208 = case shown="True" w483 {
                    tunnel: "Start Drive" -> [_ w489]
                    tunnel: w482 -> [_ w487]
                    frame False {
                    }
                    frame True {
                      n209 = Boolean To (0,1)(Boolean=w489) -> (0, 1=w488:i16)
                      n210 = To Long Integer(number=w488) -> (32bit integer=w486:i32)
                      n211 = dll-call lib="C:/Aerotech/Drivers/OGI_IF.dll" fn="StartRoadDrive"(path in=w487, "Enable"=w486) -> ()  [unwired: 2 in, 4 out]
                    }
                  }
                }
                frame #2 {
                  n212 = Not Equal?(x="Stop drive", y=w491) -> (x != y?=w495:bool)
                  n213 = Or(x=w495, y=w494) -> (x .or. y?=w493:bool)
                  n214 = case shown="True" w493 {
                    tunnel: "Stop drive" -> [_ w499]
                    tunnel: w492 -> [_ w497]
                    frame False {
                    }
                    frame True {
                      n215 = Boolean To (0,1)(Boolean=w499) -> (0, 1=w498:i16)
                      n216 = To Long Integer(number=w498) -> (32bit integer=w496:i32)
                      n217 = dll-call lib="C:/Aerotech/Drivers/OGI_IF.dll" fn="RoadStop"(path in=w497, "Enable"=w496) -> ()  [unwired: 2 in, 4 out]
                    }
                  }
                }
                frame #3 {
                  n218 = Not Equal?(x=w502, y="BL Fan2") -> (x != y?=w503:bool)
                  n219 = Not Equal?(x="BL Fan1", y=w505) -> (x != y?=w504:bool)
                  n220 = Compound Arithmetic op=OR(w504, w503, w506) -> (w507:bool)
                  n221 = case shown="True" w507 {
                    tunnel: w508 -> [_ w510]
                    tunnel: "BL Fan1" -> [_ w512]
                    tunnel: "BL Fan2" -> [_ w511]
                    frame False {
                    }
                    frame True {
                      w509 = 1 ("BL Fan (1 or 2)")
                      n222 = dll-call lib="C:/Aerotech/Drivers/OGI_IF.dll" fn="SetBoundaryPerc"(path in=w510, "enable"=w509, "BL Fan (1 or 2)"=1, "New Percentage"=w512) -> ()  [unwired: 4 in, 4 out]
                      n223 = dll-call lib="C:/Aerotech/Drivers/OGI_IF.dll" fn="SetBoundaryPerc"(path in=w510, "enable"=w509, "BL Fan (1 or 2)"=2, "New Percentage"=w511) -> ()  [unwired: 4 in, 4 out]
                    }
                  }
                }
              }
            }
          }
        }
        n224 = case shown="True" w20 {
          tunnel: [w46 w53] -> w36
          tunnel: w35 -> [_ w52]
          tunnel: w34 -> [w46 w51]
          tunnel: w33 -> [_ w50]
          tunnel: w21 -> [_ w47]
          frame False {
          }
          frame True {
            w48 = FALSE  # Give Variance
            w49 = 1.0  # Averaging Period (s)
            n225 = call "Upload_To_ADAM_Server.vi"("First Loop"=w47, "Averaging Period (s)"=w49, "Shift In"=w51, "Channel Values"=w52, "Give Variance"=w48, "Channel Names"=w50) -> ("Shift Out"=w53:dbl[])
            n226 = call "Restart_OGI_COMS.vi"() -> ()  [unwired: 12 in]
          }
        }
        n227 = node-c288() -> ()  [unwired: 1 in, 1 out]
      }
      n228 = node-c288(w15) -> ()  [unwired: 1 out]
    }
    frame #3 {
      n229 = dll-call lib="C:/Aerotech/Drivers/OGI_IF.dll" fn="CloseLink"(path in=w519) -> ()  [unwired: 2 in, 3 out]
    }
  }
